vi "Delete Platform Application.vi"(8 "error in (no error)":errorcluster, 11 "Platform Application in":refnum<class "Platform Application.lvclass">) -> (0 "error out":errorcluster)   [LabVIEW 2015, in "NI_AWS_SNS.lvlib" / "Platform Application.lvclass"]
uses:
  Platform Application.lvclass
  Core/HTTP Request/Request Options.ctl
  Core/HTTP Request/Name Value Pair.ctl
  Core/ARN/ARN.lvclass/ARN.ctl
  Core/ARN/Read ARN.vi
  Core/HTTP Request/HTTP Request.lvclass
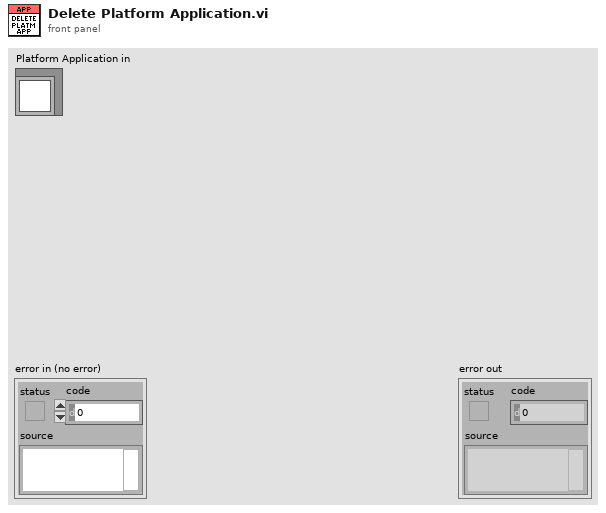
[diagram p1: front panel]
types:
  T1 = typedef "NI_AWS_Core.lvlib/HTTP Request.lvclass/Name Value Pair.ctl" = cluster{"name":string, "value":string}
  T2 = typedef "NI_AWS_Core.lvlib/HTTP Request.lvclass/Request Options.ctl" = cluster{"request headers":T1[], "request parameters":T1[], "request body":string}
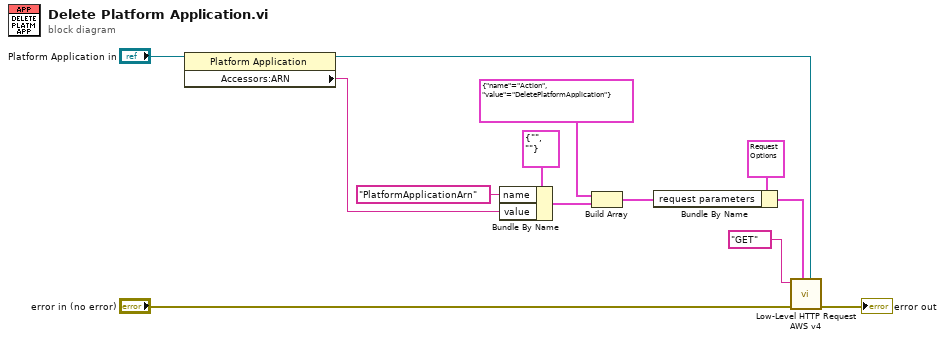
[diagram p0: block diagram]
diagram:
  n1 = property class="Platform Application"(reference="Platform Application in") -> (reference out=w2:refnum<class "Platform Application.lvclass">, "Accessors:ARN"=w1:string)  [unwired: 1 in, 1 out]
  n2 = Bundle By Name(cluster=T1 {"name"="", "value"=""} ("element"), "name"="PlatformApplicationArn", "value"=w1) -> (w7:T1)
  n3 = Build Array(T1 {"name"="Action", "value"="DeletePlatformApplication"} ("Name Value Pair"), w7) -> (w6:T1[])
  n4 = Bundle By Name(cluster=T2 {"request headers"=[], "request parameters"=[{"name"="Action", "value"="ListQueues"}], "request body"=""} ("Request Options"), "request parameters"=w6) -> (w10:T2)
  n5 = call "Low-Level HTTP Request AWS v4.vi"("AWS Core"=w2, "Request Options"=w10, "error in (no error)"="error in (no error)", "HTTP-Verb"="GET") -> ("error out"=→"error out":errorcluster)  [unwired: 5 in, 2 out]
